vi "RSZVB Set Calibration Data Default State.vi"(8 "error in (no error)":errorcluster {"code" format="%.0x"}, 9 "Keep Meas Data (F: Off)":bool, 10 "Channel (1)":i32=1, 11 "VISA session":refnum<visa-resource-name>) -> (0 "error out":errorcluster {"code" format="%.0x"}, 3 "dup VISA session":refnum<visa-resource-name>)   [LabVIEW 2011]
doc: "This VI activates or deactivates the calibration mode where the raw measurement data of the standards is stored after the calibration is completed. The setting remains valid for all subsequent calibrations until it is changed explicitly. A new calibration deletes the calibration data acquired in previous calibrations.\n\nNote(s):\n\n(1) For some measurements the default set timeout can be insufficient. To set higher timeout use VI RSZVB Set Time Out.vi.\n\nRemote-control command(s):\n[SENSe<Ch>:]CORRection:COLLect[:ACQuire]:RSAVe:DEFault <Boolean>"
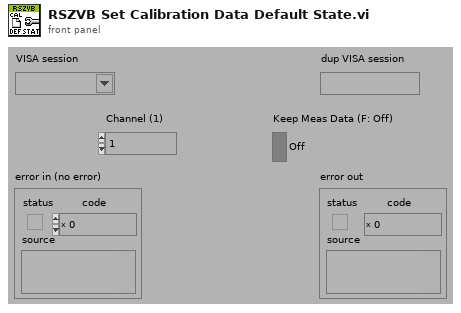
[diagram p1: front panel]
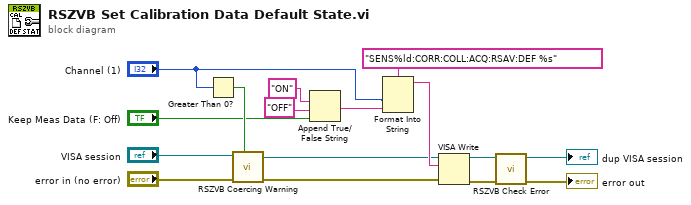
[diagram p0: block diagram]
diagram:
  n1 = Greater Than 0?(x="Channel (1)") -> (x > 0?=w9:bool)
  n2 = call "RSZVB Coercing Warning.vi"("In Range?"=w9, "error in (no error)"="error in (no error)", "VISA session"="VISA session") -> ("error out"=w8:errorcluster, "dup VISA session"=w7:refnum<visa-resource-name>)  [unwired: 7 in]
  n3 = Append True/False String(1:"Keep Meas Data (F: Off)", 2:"OFF", 3:"ON") -> (0:w10:string)  [unwired: 1 in]
  n4 = Format Into String(format string="SENS%ld:CORR:COLL:ACQ:RSAV:DEF %s", "Channel (1)", w10) -> (resulting string=w13:string)  [unwired: 2 in, 1 out]
  n5 = VISA Write(VISA resource name=w7, write buffer=w13, error in (no error)=w8) -> (VISA resource name out=w14:refnum<visa-resource-name>, error out=w15:errorcluster)  [unwired: 1 out]
  n6 = call "RSZVB Check Error.vi"("error in (no error)"=w15, "VISA session"=w14) -> ("error out"=→"error out":errorcluster, "dup VISA session"=→"dup VISA session":refnum<visa-resource-name>)  [unwired: 8 in]
